vi "updateTuplaEnDBEstadistica.vi"(8 "error in":errorcluster, 11 "claseEstadistica in":refnum<class "claseEstadistica.lvclass">) -> (0 "error out":errorcluster, 3 "claseEstadistica out":refnum<class "claseEstadistica.lvclass">)   [LabVIEW 2014, in "claseEstadistica.lvclass"]
uses:
  claseEstadistica.lvclass
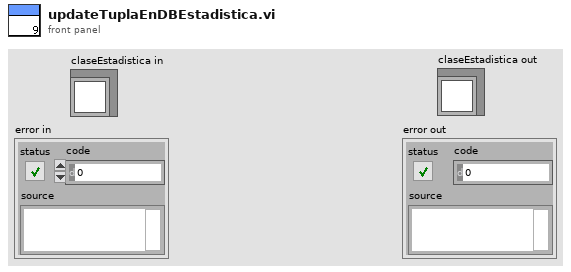
[diagram p1: front panel]
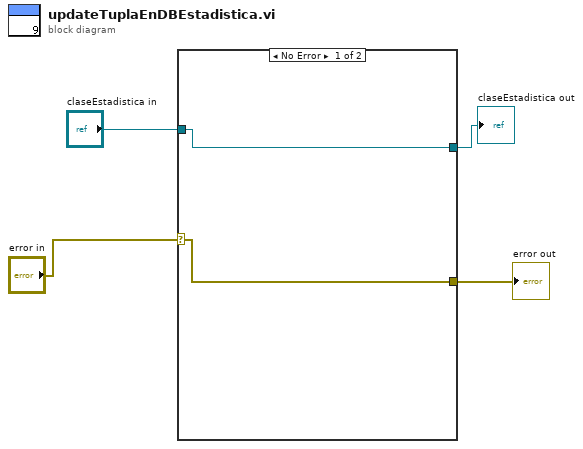
[diagram p0: block diagram]
diagram:
  n1 = case shown="No Error" "error in" {
    selector: "error in" -> [w6 w8]
    tunnel: [w6 w8] -> w3
    tunnel: [w5 w7] -> w2
    tunnel: "claseEstadistica in" -> [w5 w7]
    frame No Error {
    }
    frame Error {
    }
  }
  "claseEstadistica out" <- w2
  "error out" <- w3
